vi "Get Label Text.vi"(8 "error in (no error)":errorcluster, 11 "Control In":refnum<class "Control.lvclass">) -> (0 "error out":errorcluster, 2 "Text":string, 3 "Control Out":refnum<class "Control.lvclass">)   [LabVIEW 2017, in "Front Panel Publisher.lvlib" / "Control.lvclass"]
uses:
  Control.lvclass
  Text_class/Text.lvclass
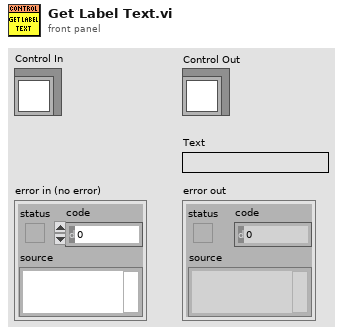
[diagram p1: front panel]
types:
  T1 = typedef "Front Panel Publisher.lvlib/Control.lvclass/Attributes.ctl" = cluster{"Description":string, "Indicator":bool, "Default Value":variant, "Control Index":i32, "Label":refnum<class "Text.lvclass">, "Caption":refnum<class "Text.lvclass">, "Image b64":string, "No Control Index":bool, "Display Mode":T2}
  T2 = typedef "Front Panel Publisher.lvlib/Web Front Panel.lvclass/Enum - Control Display Mode.ctl" = enum16{"Value Only", "Value and Visibility", "Boolean Value Only", "Boolean Value and Visibility", "Control is Image", "Image and Visibility"}
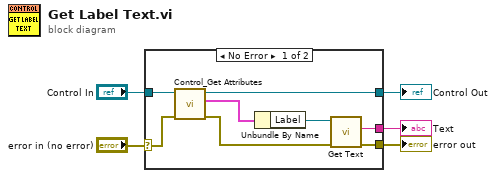
[diagram p0: block diagram]
diagram:
  n1 = case shown="No Error" "error in (no error)" {
    selector: "error in (no error)" -> [w13 w15]
    tunnel: [w7 w15] -> w4
    tunnel: [w10 w14] -> w2
    tunnel: "Control In" -> [w11 w14]
    tunnel: [w6 _] -> w1
    frame No Error {
      n2 = call "Control_Get Attributes.vi"("error in (no error)"=w13, "Control In"=w11) -> ("error out"=w8:errorcluster, "Control Attributes"=w12:T1, "Control Out"=w10:refnum<class "Control.lvclass">)  [unwired: 7 in]
      n3 = Unbundle By Name(w12) -> ("Label"=w9:refnum<class "Text.lvclass">)
      n4 = call-dynamic "Get Text.vi"("error in (no error)"=w8, "Text In"=w9) -> ("error out"=w7:errorcluster, "Text"=w6:string)  [unwired: 7 in, 1 out]
    }
    frame Error {
    }
  }
  "error out" <- w4
  "Control Out" <- w2
  "Text" <- w1
